vi "Read Attributes.vi"(11 "Set DER SetPointVF Msg":refnum<class "Set DER SetPointF Msg.lvclass">) -> (2 "Payload":cluster{"DER_SetPointF":T1})   [LabVIEW 2018, in "Device Communication and Control Abstract Actor.lvlib" / "Set DER SetPointF Msg.lvclass"]
uses:
  Set DER SetPointF Msg.lvclass
  <vilib>/ORNL/CSEISMIC DDS/CSEISMIC DDS Base/Data Types/DER_SetPointF.ctl
  <vilib>/ORNL/CSEISMIC DDS/CSEISMIC DDS Base/Data Types/Controls/DeviceID.ctl
  Set DER SetPointF Msg.lvclass/Set DER SetPointF Msg.ctl
  <vilib>/ORNL/CSEISMIC DDS/CSEISMIC DDS Base/CSEISMIC DDS.lvclass
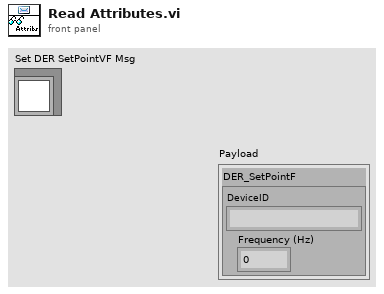
[diagram p1: front panel]
types:
  T1 = typedef "CSEISMIC DDS.lvlib/CSEISMIC DDS.lvclass/DER_SetPointF.ctl" = cluster{"DeviceID":T2, "Frequency (Hz)":dbl}
  T2 = typedef "CSEISMIC DDS.lvlib/CSEISMIC DDS.lvclass/DeviceID.ctl" = string
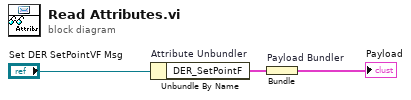
[diagram p0: block diagram]
diagram:
  n1 = Unbundle By Name "Attribute Unbundler"("Set DER SetPointVF Msg") -> ("DER_SetPointF"=w1:T1)
  n2 = Bundle "Payload Bundler"("DER_SetPointF"=w1) -> (→"Payload":cluster{"DER_SetPointF":T1})  [unwired: 1 in]
